vi "complete_tour.vi"(3 "core_data in":T1) -> (0 "the recently completed tour":T6, 1 "core_data out":T1)   [LabVIEW 2020, in "core.lvlib"]
uses:
  core.lvlib
  core_data/completed_tour.ctl
  core_data/chessboard_index.ctl
  core_data/tour type (enum).ctl
  core_data/core_data.ctl
  core_data/tour_in_progress.ctl
  core_data/chess_square.ctl
  core_data/neighbour_square.ctl
  core_data/core_data.lvlib
panel:
  # "Development\ncontrols/indicators useful for development and testing, but which are not outputs of the VI"
  # "Input\nInputs to the VI"
  # "Output\nOutputs of the VI"
  # "Description\n\nBlank VI with error handling case. \n\nSummarize the use of this VI in this space."
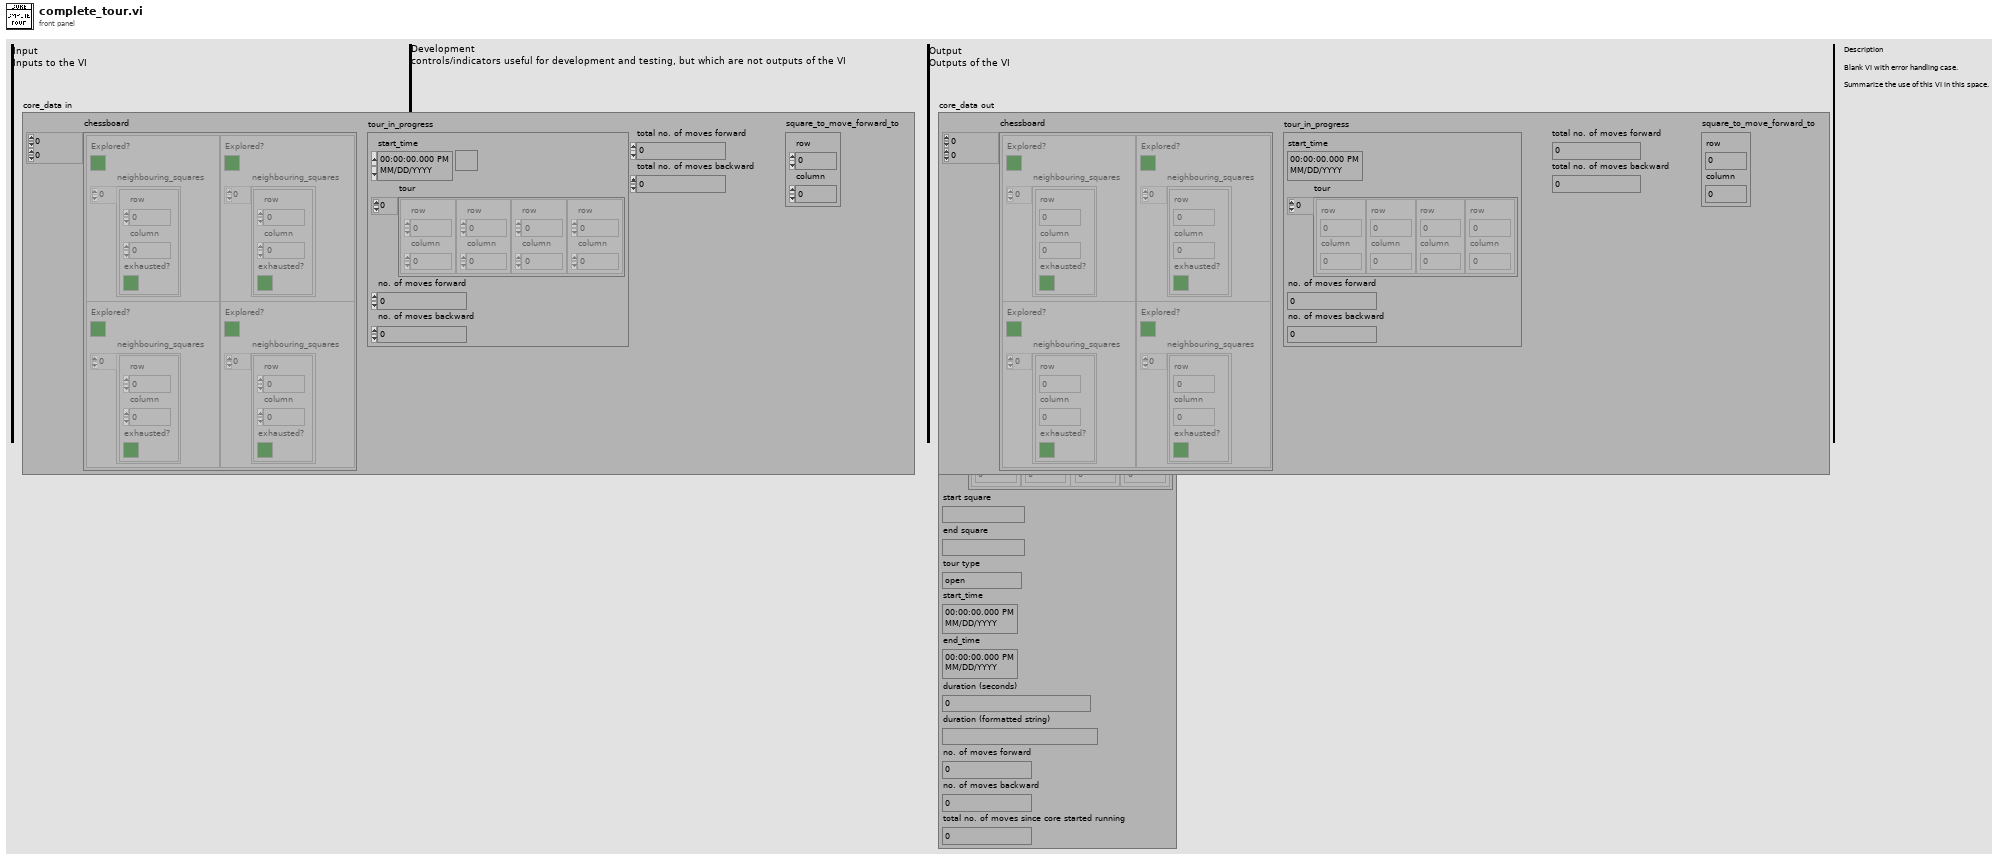
[diagram p1: front panel]
types:
  T1 = typedef "core.lvlib/core_data.lvlib/core_data.ctl" = cluster{"tour_in_progress":T2, "total no. of moves forward":u64, "total no. of moves backward":u64, "chessboard":T4[][], "square_to_move_forward_to":T3}
  T2 = typedef "core.lvlib/core_data.lvlib/tour_in_progress.ctl" = cluster{"start_time":timestamp, "tour":T3[], "no. of moves forward":u64, "no. of moves backward":u64}
  T3 = typedef "core.lvlib/core_data.lvlib/chessboard_index.ctl" = cluster{"row":u8, "column":u8}
  T4 = typedef "core.lvlib/core_data.lvlib/chess_square.ctl" = cluster{"Explored?":bool, "neighbouring_squares":T5[]}
  T5 = typedef "core.lvlib/core_data.lvlib/neighbour_square.ctl" = cluster{"row":u8, "column":u8, "exhausted?":bool}
  T6 = typedef "core.lvlib/core_data.lvlib/completed_tour.ctl" = cluster{"complete_tour":T3[], "start square":string, "end square":string, "tour type":T7, "start_time":timestamp, "end_time":timestamp, "duration (seconds)":dbl, "duration (formatted string)":string, "no. of moves forward":u64, "no. of moves backward":u64, "total no. of moves since core started running":u64}
  T7 = typedef "core.lvlib/core_data.lvlib/tour type (enum).ctl" = enum16{"open", "closed"}
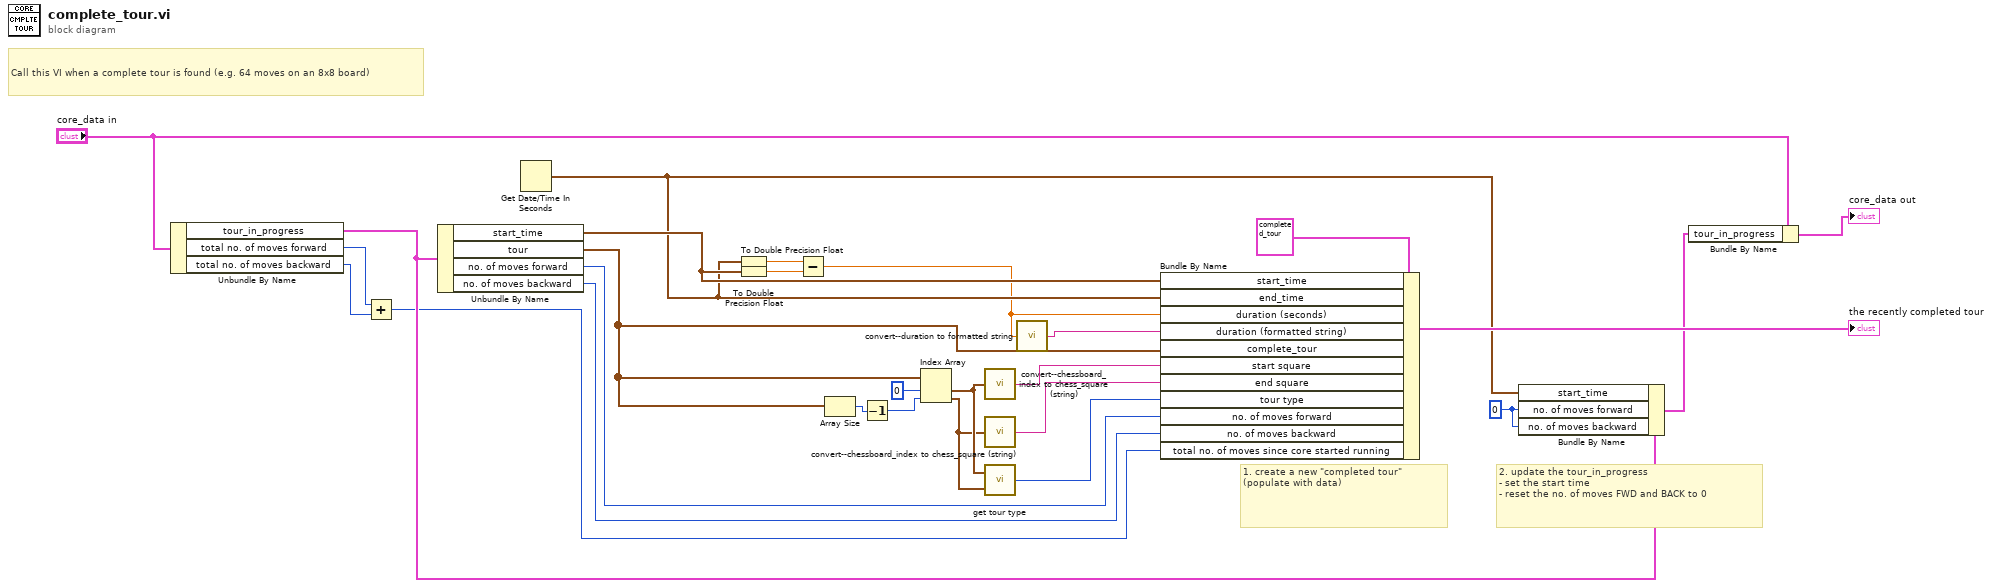
[diagram p0: block diagram]
diagram:
  w14 = u64 0 ("no. of moves forward")
  # "2. update the tour_in_progress\n- set the start time\n- reset the no. of moves FWD and BACK to 0"
  # "1. create a new \"completed tour\" (populate with data)"
  # "Call this VI when a complete tour is found (e.g. 64 moves on an 8x8 board)"
  n1 = Unbundle By Name("core_data in") -> ("tour_in_progress"=w17:T2, "total no. of moves forward"=w3:u64, "total no. of moves backward"=w2:u64)
  n2 = Add(x=w3, y=w2) -> (x+y=w1:u64)
  n3 = Unbundle By Name(w17) -> ("start_time"=w23:timestamp, "tour"=w13:T3[], "no. of moves forward"=w5:u64, "no. of moves backward"=w4:u64)
  n4 = Get Date/Time In Seconds() -> (seconds since 1Jan1904=w15:timestamp)
  n5 = To Double Precision Float(number=w15) -> (double precision float=w22:dbl)
  n6 = To Double Precision Float(number=w23) -> (double precision float=w21:dbl)
  n7 = Subtract(x=w22, y=w21) -> (x-y=w12:dbl)
  n8 = Array Size(array=w13) -> (size(s)=w19:i32)
  n9 = Decrement(x=w19) -> (x-1=w18:i32)
  n10 = Index Array(array=w13, index #1=0 ("index"), index #2=w18) -> (element #1=w8:T3, element #2=w7:T3)
  n11 = call "convert--chessboard_index to chess_square (string).vi"("chessboard_index"=w8) -> ("chess square (string)"=w10:string)
  n12 = call "convert--chessboard_index to chess_square (string).vi"("chessboard_index"=w7) -> ("chess square (string)"=w9:string)
  n13 = call "get tour type.vi"("end square"=w7, "start square"=w8) -> ("tour type"=w6:T7)
  n14 = call "convert--duration to formatted string.vi"("duration (seconds)"=w12) -> ("duration (formatted string)"=w11:string)
  n15 = Bundle By Name(cluster=T6 {"complete_tour"=[], "start square"="", "end square"="", "tour type"=enum."open", "start_time"=timestamp(0 s since 1904-01-01), "end_time"=timestamp(0 s since 1904-01-01), "duration (seconds)"=0.0, "duration (formatted string)"="", "no. of moves forward"=0, "no. of moves backward"=0, "total no. of moves since core started running"=0} ("completed_tour"), "start_time"=w23, "end_time"=w15, "duration (seconds)"=w12, "duration (formatted string)"=w11, "complete_tour"=w13, "start square"=w10, "end square"=w9, "tour type"=w6, "no. of moves forward"=w5, "no. of moves backward"=w4, "total no. of moves since core started running"=w1) -> (→"the recently completed tour":T6)
  n16 = Bundle By Name(cluster=w17, "start_time"=w15, "no. of moves forward"=w14, "no. of moves backward"=w14) -> (w16:T2)
  n17 = Bundle By Name(cluster="core_data in", "tour_in_progress"=w16) -> (→"core_data out":T1)
